vi "WGP3.vi"(0 "Header Comments":string="This is a C(T) experiment being done in Physics 350.\r\nIt records the decay response of an RC circuit where the capacitance is a strong function of temperature.", 11 "error in":errorcluster) -> (3 "Proceed":bool, 4 "data file path out":path, 10 "Timing Control Parameters out":T1={"N cycles for averaging"=3, "N points per measurment"=3, "Measurment time interval"=3.0} {"Measurment time interval" format="%.2e"}, 14 "Auto Launch Data Viewer at End":bool=TRUE, 15 "error out":errorcluster)   [LabVIEW 2017]
uses:
  typedefs/time control params.ctl
  typedefs/temp control params.ctl
panel:
  in  "N temps":i32=6
  in  "time control parameters":T1={"N cycles for averaging"=10, "N points per measurment"=1000, "Measurment time interval"=2e-05} {"Measurment time interval" format="%.2e"}
  in  "temp control parameters":T2={"Start Temp"=30.0, "Temp Step"=10.0, "End Temp"=80.0} {"End Temp" format="%.2f"; "Temp Step" format="%.2f"; "Start Temp" format="%.2f"}
  out "Temp Array":dbl[](array[numeric])=[3.0]
  in  "reload parameters":bool
  in  "exit":bool
  in  "create file and proceed":bool
  out "File Header":string="This is a C(T) experiment being done in Physics 350.\r\nIt records the decay response of an RC circuit where the capacitance is a strong function of temperature.\n\nStart temp = 3.000000\nTemp step = 3.000000\nEnd temp = 3.000000\nNum temps = 5\nNum avg cycles = 3\nNum points per meas = 3\nMeas time interval = 3.000000E+0\n\n<data below>\n\n"
  in  "Auto Launch Data Viewer at End":bool=TRUE
  # "P350 C(T) Experimental Initialization"
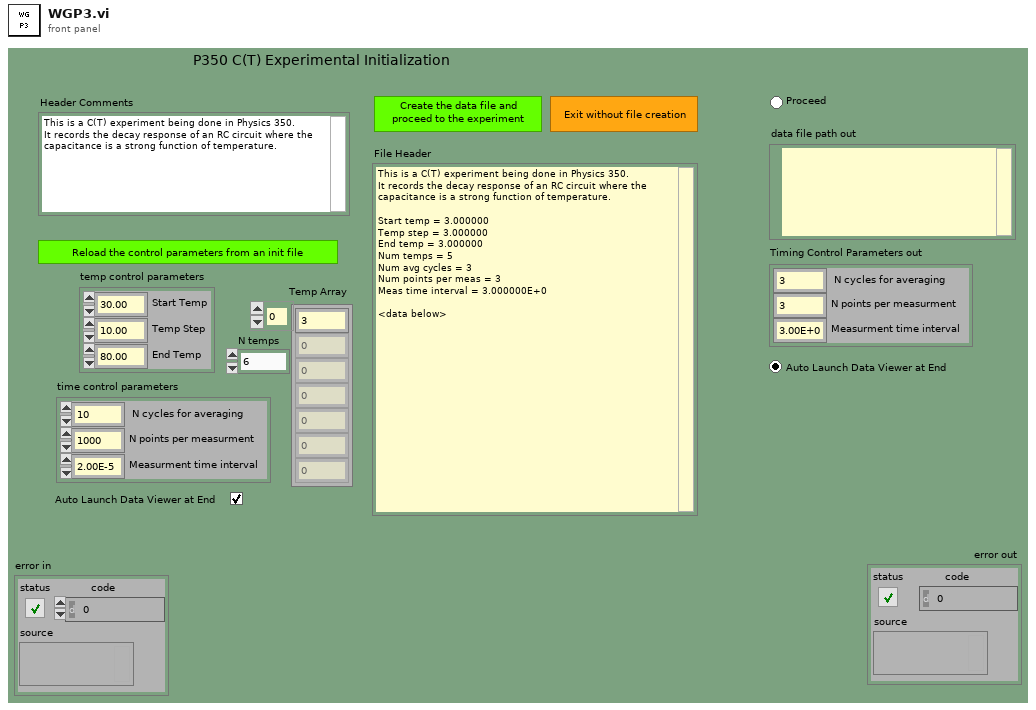
[diagram p1: front panel]
types:
  T1 = typedef "time control params.ctl" = cluster{"N cycles for averaging":i32, "N points per measurment":i32, "Measurment time interval":dbl}
  T2 = typedef "temp control params.ctl" = cluster{"Start Temp":dbl, "Temp Step":dbl, "End Temp":dbl}
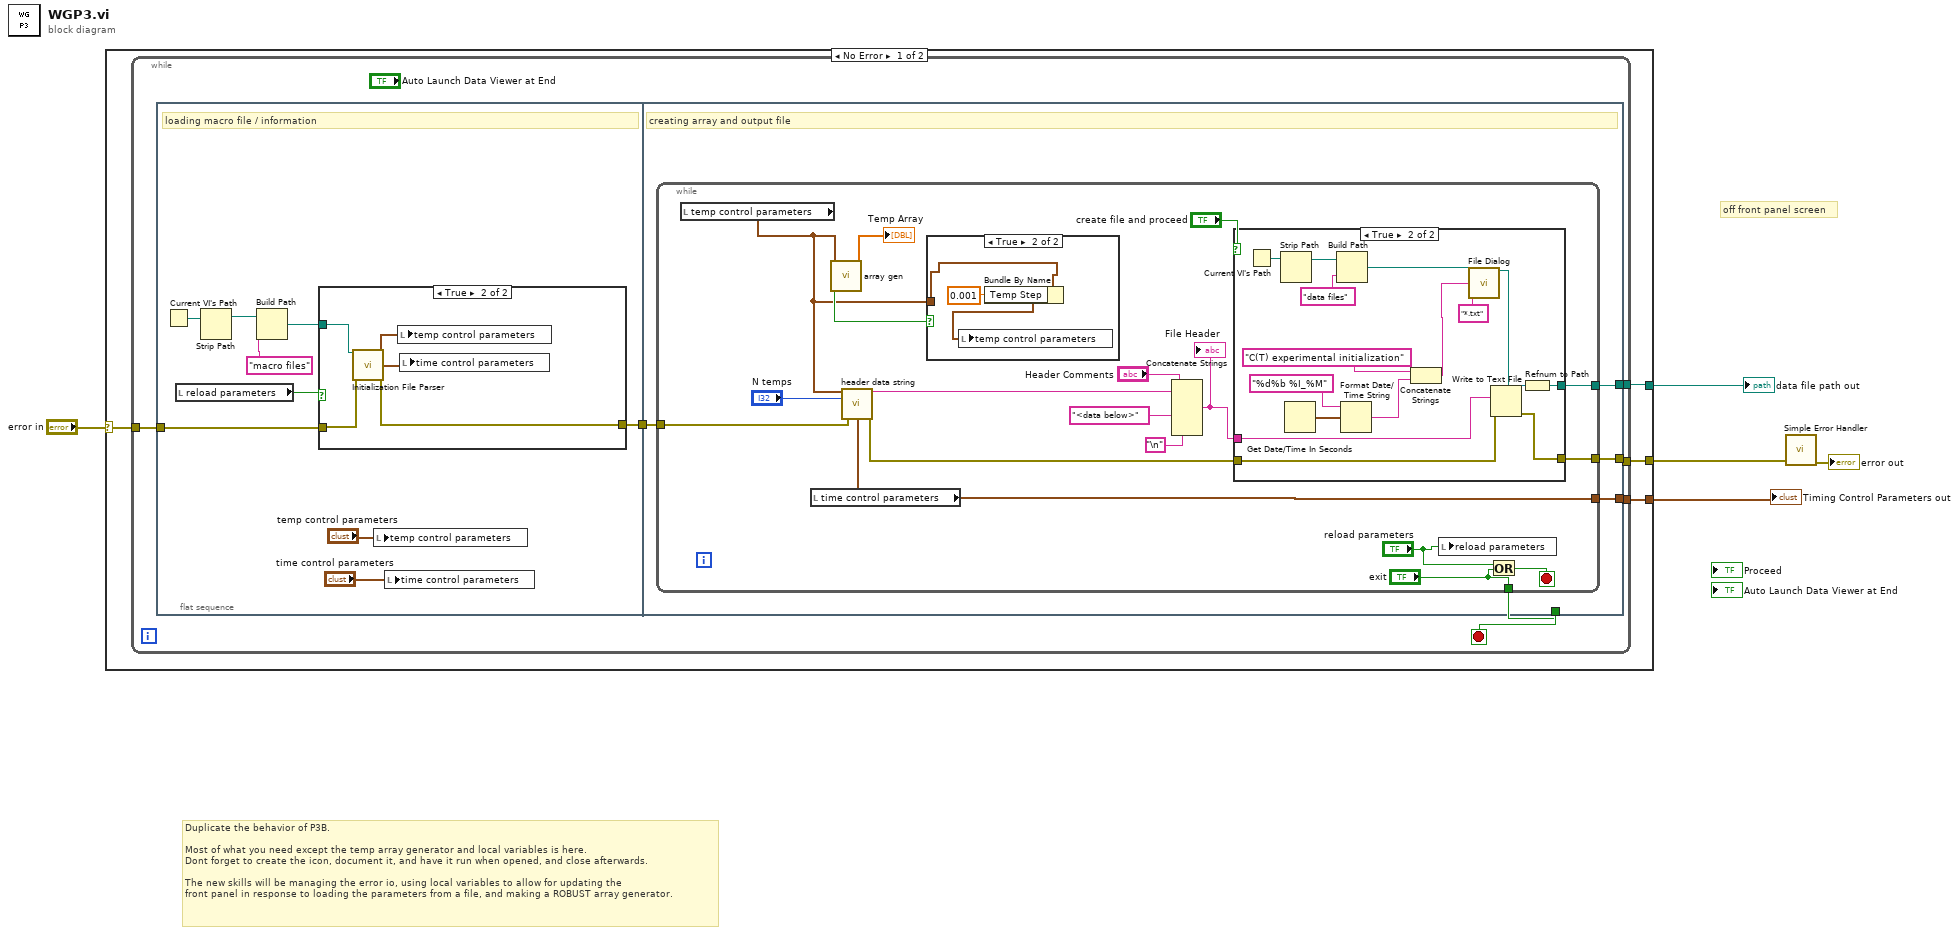
[diagram p0: block diagram]
diagram:
  # "off front panel screen"
  # "Duplicate the behavior of P3B.\n\nMost of what you need except the temp array generator and local variables is here. \nDont forget to create the icon, document it, and have it run when opened, and close afterwards.\n\nThe new skills will be managing the error io, using local variables to allow for updating the\nfront panel in response to loading the parameters from a file, and making a ROBUST array generator."
  n1 = case shown="No Error" "error in" {
    selector: "error in" -> [w9 w74]
    tunnel: [w7 w74] -> w2
    tunnel: [w8 _] -> w3
    tunnel: [w6 _] -> w1
    frame No Error {
      n2 = while {
        tunnel: [w14] -> w8
        tunnel: [w12] -> w6
        tunnel: w9 -> [w15]
        tunnel: [w13] -> w7
        stop <- w11 stop-if-true
        n3 = flat-sequence {
          tunnel: w15 -> [w24]
          tunnel: [w23] -> w10
          tunnel: w10 -> [w31]
          tunnel: [w32] -> w14
          tunnel: [w35] -> w12
          tunnel: [w34] -> w13
          tunnel: [w33] -> w11
          frame #0 {
            # "loading macro file / information"
            n4 = Current VI's Path() -> (path=w20:path)
            n5 = local read "reload parameters"() -> (w22:bool)
            n6 = Strip Path(path=w20) -> (stripped path=w21:path)  [unwired: 1 out]
            n7 = Build Path(base path=w21, name or relative path="macro files") -> (appended path=w18:path)
            n8 = case shown="True" w22 {
              tunnel: w24 -> [w25 w30]
              tunnel: [w25 w29] -> w23
              tunnel: w18 -> [_ w26]
              frame False {
              }
              frame True {
                n9 = call "Initialization File Parser.vi"("path in"=w26, "error in"=w30) -> ("temp control parameters"=w28:T2, "time control parameters"=w27:T1, "error out"=w29:errorcluster)  [unwired: 9 in, 2 out]
                n10 = local write "temp control parameters"(w28) -> ()
                n11 = local write "time control parameters"(w27) -> ()
              }
            }
            n12 = local write "temp control parameters"("temp control parameters") -> ()
            n13 = local write "time control parameters"("time control parameters") -> ()
          }
          frame #1 {
            # "creating array and output file"
            n14 = while {
              tunnel: [w53] -> w35
              tunnel: [w52] -> w34
              tunnel: ["exit"] -> w33
              tunnel: [w39] -> w32
              tunnel: w31 -> [w38]
              stop <- w50 stop-if-true
              w46 = "\n"
              n15 = local read "temp control parameters"() -> (w36:T2)
              n16 = local read "time control parameters"() -> (w39:T1)
              n17 = call "array gen.vi"("Temperature Control Parameters"=w36) -> ("Temp Array"=→"Temp Array":dbl[], "too low"=w37:bool)  [unwired: 9 in]
              n18 = call "header data string.vi"("Temperature Control Parameters"=w36, "N temps"="N temps", "error in (no error)"=w38, "Timing Control Parameters"=w39) -> ("Header string component"=w41:string, "error out"=w40:errorcluster)  [unwired: 10 in]
              n19 = case shown="True" w37 {
                tunnel: w36 -> [_ w56]
                frame False {
                }
                frame True {
                  n20 = Bundle By Name(cluster=w56, "Temp Step"=0.001) -> (w55:T2)
                  n21 = local write "temp control parameters"(w55) -> ()
                }
              }
              n22 = Concatenate Strings("Header Comments", w41, w46, w46, "<data below>", w46, w46) -> (w44:string)
              "File Header" <- w44
              n23 = case shown="True" "create file and proceed" {
                tunnel: w44 -> [_ w73]
                tunnel: [_ w71] -> w53
                tunnel: w40 -> [w57 w70]
                tunnel: [w57 w69] -> w52
                frame False {
                }
                frame True {
                  n24 = Current VI's Path() -> (path=w67:path)
                  n25 = Strip Path(path=w67) -> (stripped path=w68:path)  [unwired: 1 out]
                  n26 = Get Date/Time In Seconds() -> (seconds since 1Jan1904=w60:timestamp)
                  n27 = Build Path(base path=w68, name or relative path="data files") -> (appended path=w65:path)
                  n28 = Format Date/Time String(time format string (%c)="%d%b %I_%M", seconds (now)=w60) -> (date/time string=w59:string)  [unwired: 1 in]
                  n29 = Concatenate Strings("C(T) experimental initialization", w59) -> (w61:string)
                  n30 = call "File Dialog"("start path"=w65, "default name"=w61, "pattern (all files)"="*.txt") -> ("selected path"=w64:path)  [unwired: 9 in, 3 out]
                  n31 = Write to Text File(file (use dialog)=w64, text=w73, error in=w70) -> (refnum out=w72:refnum<file>, error out=w69:errorcluster)  [unwired: 1 in, 1 out]
                  n32 = Refnum to Path(1:w72) -> (0:w71:path)
                }
              }
              n33 = local write "reload parameters"("reload parameters") -> ()
              n34 = Or(x="reload parameters", y="exit") -> (x .or. y?=w50:bool)
            }
          }
        }
      }
    }
    frame Error {
    }
  }
  "Timing Control Parameters out" <- w3
  "data file path out" <- w1
  n35 = call <vilib>:"Simple Error Handler.vi"("error in (no error)"=w2) -> ("error out"=→"error out":errorcluster)  [unwired: 4 in, 4 out]
